vi "Write Header parameters 2.vi"(8 "error in (no error)":errorcluster, 10 "Header parameters":T1={"COMNENT"="", "OBSTYPE"="OBJECT", "ACSVRSN"="", "CHANNEL"=0, "LAST_IMG_NAME"="", "NIGHTDIR"="E:\\images\\today\\"}, 11 "Save Image in":refnum<class "Save Image.lvclass">) -> (0 "error out":errorcluster, 3 "Save Image out":refnum<class "Save Image.lvclass">)   [LabVIEW 2018, in "Save Image.lvclass"]
uses:
  Save Image.lvclass
  Save Image.lvclass/Save Image.ctl
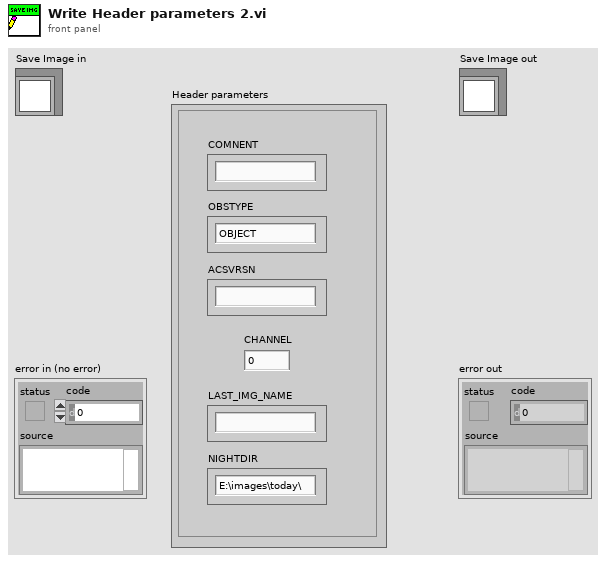
[diagram p1: front panel]
types:
  T1 = cluster{"COMNENT":string, "OBSTYPE":string, "ACSVRSN":string, "CHANNEL":u16, "LAST_IMG_NAME":string, "NIGHTDIR":string}
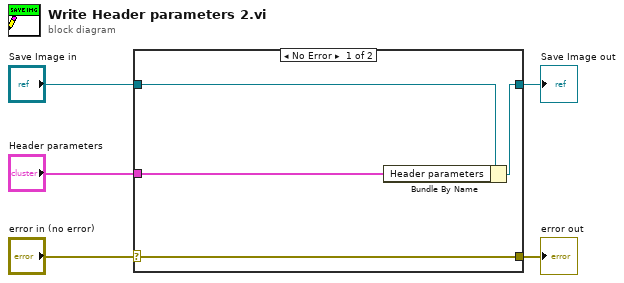
[diagram p0: block diagram]
diagram:
  n1 = case shown="No Error" "error in (no error)" {
    selector: "error in (no error)" -> [w9 w10]
    tunnel: [w9 w10] -> w4
    tunnel: [w7 w11] -> w2
    tunnel: "Save Image in" -> [w8 w11]
    tunnel: "Header parameters" -> [w6 _]
    frame No Error {
      n2 = Bundle By Name(cluster=w8, "Header parameters"=w6) -> (w7:refnum<class "Save Image.lvclass">)
    }
    frame Error {
    }
  }
  "error out" <- w4
  "Save Image out" <- w2
